vi "Add DIO card.vi"(8 "error in (no error)":errorcluster, 11 "Node Ptr":u64 format="%.0x") -> (0 "error out":errorcluster)   [LabVIEW 2014, in "SLSC configuration System Explorer.lvlib"]
uses:
  Shared/Constants.vi
  <vilib>/NI Veristand/Custom Device API/Set Item Property (Variant).vi
  SLSC configuration System Explorer.lvlib
  <vilib>/NI Veristand/Custom Device API/Custom Device API.lvlib
  Shared/SLSC configuration Shared.lvlib
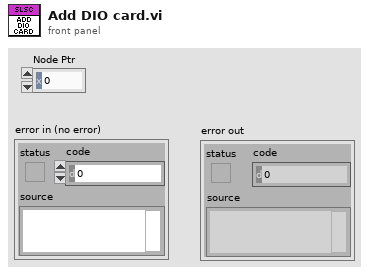
[diagram p1: front panel]
types:
  T1 = typedef "SLSC configuration Shared.lvlib/Card Postion.ctl" = cluster{"Chassis #":u8, "Slot #":u8}
  T2 = typedef "Custom Device API.lvlib/Custom Device Item Ref.ctl" = u64
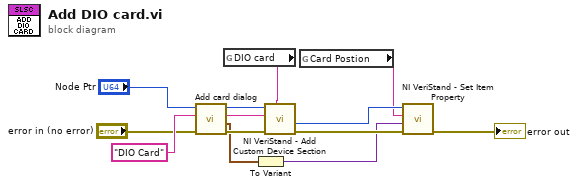
[diagram p0: block diagram]
diagram:
  n1 = call "Add card dialog.vi"("error in (no error)"="error in (no error)", "Card Type in"="DIO Card" ("Section Name"), "Node Ptr"="Node Ptr") -> ("error out"=w8:errorcluster, "Card position out"=w3:T1, "Name out"=w7:string, "Node Ptr out"=w6:u64)  [unwired: 4 in, 1 out]
  n2 = global read "Constants.vi" "DIO card"() -> (w12:string)
  n3 = To Variant(anything=w3) -> (Variant=w2:variant)
  n4 = call <vilib>:"NI VeriStand - Add Custom Device Section.vi"("GUID (Default Section)"=w12, "error in (no error)"=w8, "Section Name"=w7, "Parent Ref in"=w6) -> ("error out"=w13:errorcluster, "Section Ptr"=w4:T2)  [unwired: 4 in, 2 out]
  n5 = global read "Constants.vi" "Card Postion"() -> (w1:string)
  n6 = call-poly <vilib>:"NI VeriStand - Set Item Property.vi"("error in (no error)"=w13, "Value"=w2, "Property Name"=w1, "Item Ref in"=w4) -> ("error out"=→"error out":errorcluster)  [unwired: 5 in, 2 out]
